vi "File_IO.vi"(7 "File Enum":T1, 8 "error in (no error)":errorcluster, 10 "Total Cups In":i32, 11 "Shutdown? In":bool) -> (0 "error out":errorcluster, 2 "Total Cups Out":i32, 3 "Shutdown? Out":bool)   [LabVIEW 2026]
doc: "Read and write to the Coffee.in file which holds data related to a proper shutdown and total cups of coffee."
uses:
  controls/File_Enum.ctl
  <vilib>/Utility/config.llb/Read Key (Boolean).vi
  <vilib>/Utility/config.llb/Read Key (I32).vi
  <vilib>/Utility/config.llb/Write Key (Boolean).vi
  <vilib>/Utility/config.llb/Write Key (I32).vi
  <vilib>/Utility/config.llb/NI_LVConfig.lvlib
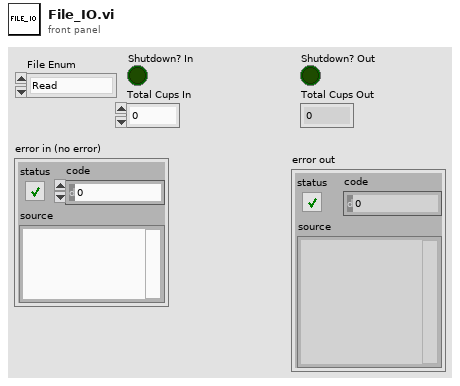
[diagram p1: front panel]
types:
  T1 = typedef "File_Enum.ctl" = enum16{"Read", "Write", "Close"}
  T2 = typedef "NI_LVConfig.lvlib/Config Data RefNum.ctl" = refnum<k1>
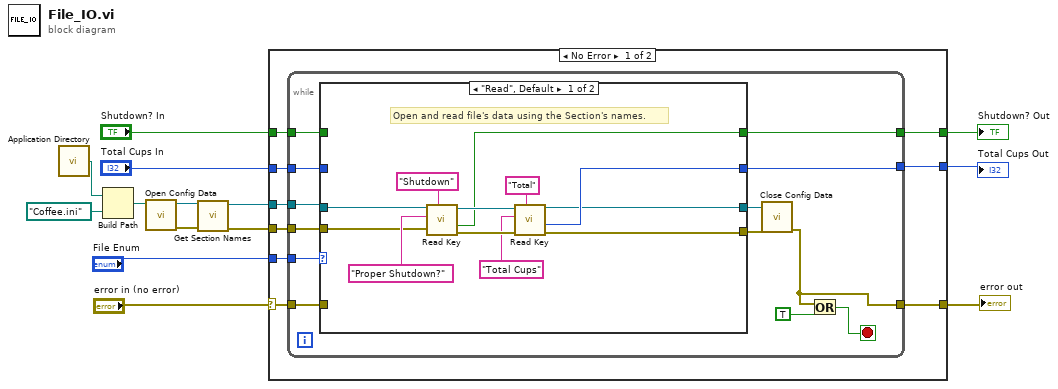
[diagram p0: block diagram]
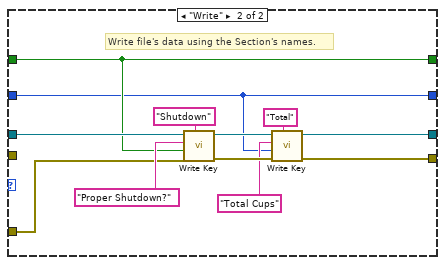
[diagram p2: hidden frame]
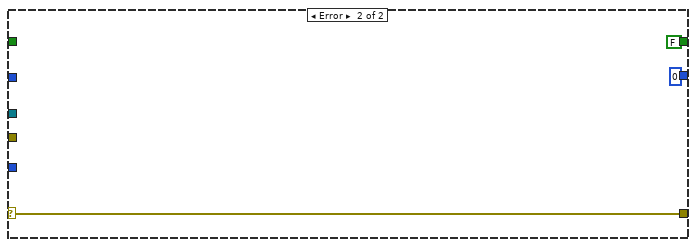
[diagram p3: hidden frame]
diagram:
  n1 = call <vilib>:"Application Directory.vi"() -> ("Application Directory"=w7:path)
  n2 = Build Path(base path=w7, name or relative path=path "Coffee.ini") -> (appended path=w6:path)
  n3 = call <vilib>:"Open Config Data.vi"("configuration file path"=w6) -> ("error out"=w4:errorcluster, "refnum"=w5:T2)  [unwired: 8 in, 1 out]
  n4 = call <vilib>:"Get Section Names.vi"("error in (no error)"=w4, "refnum"=w5) -> ("error out"=w1:errorcluster, "refnum out"=w2:T2)  [unwired: 7 in, 1 out]
  n5 = case shown="No Error" "error in (no error)" {
    selector: "error in (no error)" -> [w20 w61]
    tunnel: "File Enum" -> [w23 _]
    tunnel: [w22 FALSE ("value")] -> w13
    tunnel: [w21 0 ("value")] -> w12
    tunnel: [w19 w61] -> w10
    tunnel: "Shutdown? In" -> [w18 _]
    tunnel: "Total Cups In" -> [w17 _]
    tunnel: w2 -> [w15 _]
    tunnel: w1 -> [w16 _]
    frame No Error {
      n6 = while {
        tunnel: w23 -> [w36]
        tunnel: [w35] -> w22
        tunnel: [w34] -> w21
        tunnel: w20 -> [w33]
        tunnel: [w25] -> w19
        tunnel: w18 -> [w30]
        tunnel: w17 -> [w29]
        tunnel: w16 -> [w28]
        tunnel: w15 -> [w24]
        stop <- w31 stop-if-true
        n7 = case shown="\"Read\", Default" w36 {
          tunnel: [w44 w51] -> w35
          tunnel: [w43 w50] -> w34
          tunnel: [w42 w56] -> w27
          tunnel: w24 -> [w37 w52]
          tunnel: w33 -> [_ w53]
          tunnel: w30 -> [_ w51]
          tunnel: w29 -> [_ w50]
          tunnel: w28 -> [w39 _]
          tunnel: [w38 w49] -> w26
          frame "Read", Default {
            # "Open and read file's data using the Section's names."
            n8 = call-poly <vilib>:"Read Key.vi"("section"="Shutdown", "error in (no error)"=w39, "key"="Proper Shutdown?", "refnum"=w37) -> ("error out"=w45:errorcluster, "value"=w44:bool, "refnum out"=w48:T2)  [unwired: 4 in, 1 out]
            n9 = call-poly <vilib>:"Read Key.vi"("section"="Total", "error in (no error)"=w45, "key"="Total Cups", "refnum"=w48) -> ("error out"=w38:errorcluster, "value"=w43:i32, "refnum out"=w42:T2)  [unwired: 4 in, 1 out]
          }
          frame "Write" {
            # "Write file's data using the Section's names."
            n10 = call-poly <vilib>:"Write Key.vi"("section"="Shutdown", "error in (no error)"=w53, "value"=w51, "key"="Proper Shutdown?", "refnum"=w52) -> ("error out"=w57:errorcluster, "refnum out"=w60:T2)  [unwired: 4 in, 1 out]
            n11 = call-poly <vilib>:"Write Key.vi"("section"="Total", "error in (no error)"=w57, "value"=w50, "key"="Total Cups", "refnum"=w60) -> ("error out"=w49:errorcluster, "refnum out"=w56:T2)  [unwired: 4 in, 1 out]
          }
        }
        n12 = call <vilib>:"Close Config Data.vi"("error in (no error)"=w26, "refnum"=w27) -> ("error out"=w25:errorcluster)  [unwired: 8 in, 1 out]
        n13 = Or(x=w25, y=TRUE) -> (x .or. y?=w31:bool)
      }
    }
    frame Error {
    }
  }
  "Shutdown? Out" <- w13
  "Total Cups Out" <- w12
  "error out" <- w10
